vi "Update Value.vi"(6 "Time":dbl, 8 "error in (no error)":errorcluster, 11 "DblNumericStatusIndicator in":refnum<class "DblStatusIndicator.lvclass">) -> (0 "error out":errorcluster, 1 "Update":bool, 2 "Value":variant, 3 "DblNumericStatusIndicator out":refnum<class "DblStatusIndicator.lvclass">)   [LabVIEW 2023, in "VolatusGUIElements.lvlib" / "DblStatusIndicator.lvclass"]
uses:
  DblStatusIndicator.lvclass
  DblStatusIndicator.lvclass/DblStatusIndicator.ctl
  lv-vecto/Vecto/Channel DBL/Channel DBL.lvclass/Channel DBL.ctl
  lv-vecto/Vecto/Group DBL/Value by Index.vi
  lv-vecto/Vecto/Channel DBL/Channel DBL.lvclass
panel:
  out "Age":dbl format="%<%H:%M:%S%3u>t"
  out "Timestamp":dbl format="%<%H:%M:%S%3u\n%Y/%m/%d>T"
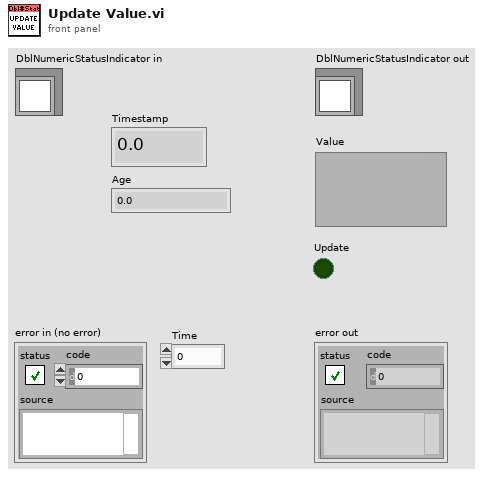
[diagram p1: front panel]
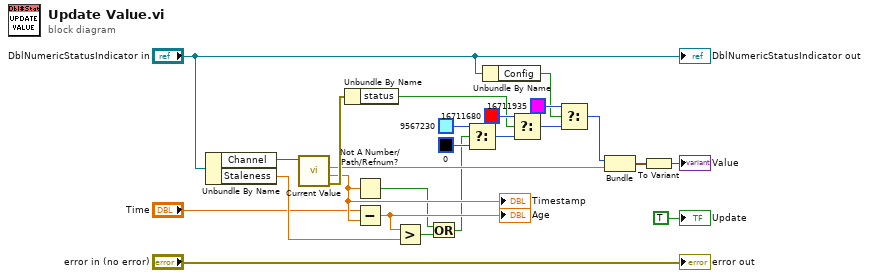
[diagram p0: block diagram]
diagram:
  n1 = Unbundle By Name("DblNumericStatusIndicator in") -> ("Channel"=w22:refnum<class "Channel DBL.lvclass">, "Staleness"=w14:dbl)
  n2 = call "Current Value.vi"("Channel in"=w22) -> ("error out"=w24:errorcluster, "Timestamp"=w13:dbl, "Scaled"=w21:dbl)  [unwired: 6 in, 2 out]
  "Timestamp" <- w13
  n3 = Unbundle By Name(w24) -> ("status"=w5:bool)
  n4 = Not A Number/Path/Refnum?(number/path/refnum=w13) -> (NaN/Path/Refnum?=w11:bool)
  n5 = Subtract(x="Time", y=w13) -> (x-y=w15:dbl)
  "Age" <- w15
  n6 = Greater?(x=w15, y=w14) -> (0:w18:bool)
  n7 = Or(x=w11, y=w18) -> (x .or. y?=w12:bool)
  n8 = Select(t=u32 9567230, s=w12, f=u32 0) -> (s? t:f=w7:u32)
  n9 = Unbundle By Name("DblNumericStatusIndicator in") -> ("Config"=w2:bool)
  n10 = Select(t=u32 16711680, s=w5, f=w7) -> (s? t:f=w4:u32)
  n11 = Select(t=u32 16711935, s=w2, f=w4) -> (s? t:f=w1:u32)
  n12 = Bundle(w1, "Scaled"=w21) -> (w17:cluster{u32, "Scaled":dbl})  [unwired: 1 in]
  n13 = To Variant(anything=w17) -> (Variant=→"Value":variant)
  "error out" <- "error in (no error)"
  "DblNumericStatusIndicator out" <- "DblNumericStatusIndicator in"
  "Update" <- TRUE ("Update")
